vi "SetConfig.vi"(8 "error in (no error)":errorcluster, 10 "Variant":variant, 11 "FunctionBase in":refnum<class "FunctionBase.lvclass">) -> (0 "error out":errorcluster, 3 "FunctionBase out":refnum<class "FunctionBase.lvclass">)   [LabVIEW 2014, in "Functions.lvlib" / "FunctionBase.lvclass"]
uses:
  FunctionBase.lvclass
  <userlib>/NIST/BaseClasses/Object_class/BaseObject.lvclass
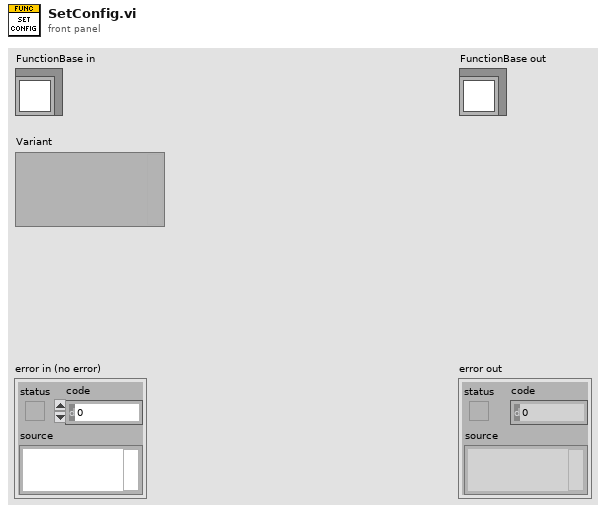
[diagram p1: front panel]
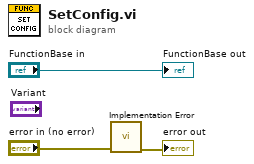
[diagram p0: block diagram]
diagram:
  n1 = call <userlib>:"Implementation Error.vi"("error in (no error)"="error in (no error)") -> ("error out"=→"error out":errorcluster)  [unwired: 10 in]
  "FunctionBase out" <- "FunctionBase in"
